vi "xps_panel_generate_abort_move_queue.vi"(8 "error in (no error)":errorcluster, 11 "newport_xps_panel in":refnum<class "newport_xps_panel.lvclass">) -> (0 "error out":errorcluster, 3 "newport_xps_panel out":refnum<class "newport_xps_panel.lvclass">)   [LabVIEW 2015, in "newport_xps_panel.lvclass"]
uses:
  newport_xps_panel.lvclass
  newport_xps_panel.lvclass/newport_xps_panel.ctl
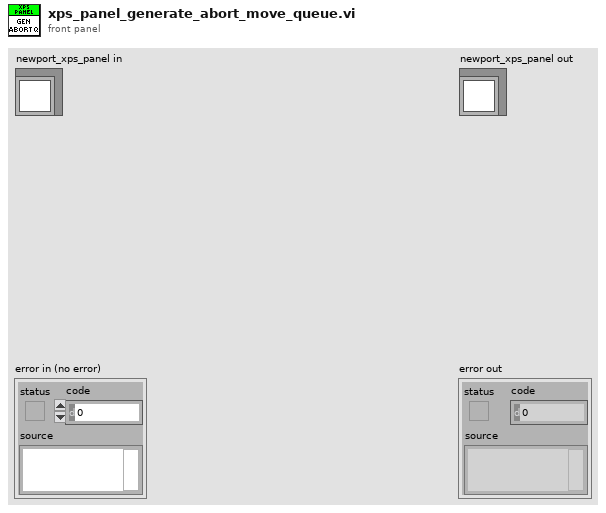
[diagram p1: front panel]
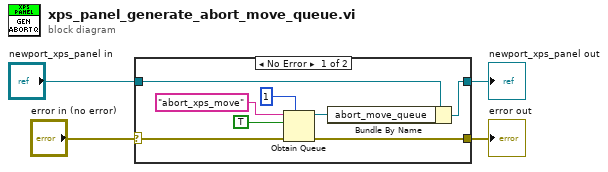
[diagram p0: block diagram]
diagram:
  n1 = case shown="No Error" "error in (no error)" {
    selector: "error in (no error)" -> [w9 w14]
    tunnel: [w5 w14] -> w3
    tunnel: [w6 w13] -> w1
    tunnel: "newport_xps_panel in" -> [w7 w13]
    frame No Error {
      n2 = Obtain Queue(max queue size (-1, unlimited)=1, name (unnamed)="abort_xps_move", element data type=TRUE, error in (no error)=w9) -> (queue out=w8:refnum<queue>, error out=w5:errorcluster)  [unwired: 1 in, 1 out]
      n3 = Bundle By Name(cluster=w7, "abort_move_queue"=w8) -> (w6:refnum<class "newport_xps_panel.lvclass">)
    }
    frame Error {
    }
  }
  "error out" <- w3
  "newport_xps_panel out" <- w1
